vi "Get Module Configuration Example.vi"() -> ()   [LabVIEW 2017]
uses:
  <userlib>/_NEVSTOP/Communicable State Machine(CSM)/_Support/Priority Queue/Priority Queue.lvclass/Priority Queue.ctl
  <userlib>/_NEVSTOP/Communicable State Machine(CSM)/_Support/Process/CSMP-Sync Call.vi
  <userlib>/_NEVSTOP/Communicable State Machine(CSM)/Utility/uuid.vi
  <userlib>/_NEVSTOP/Communicable State Machine(CSM)/Utility/Build Error Cluster.vi
  <userlib>/_NEVSTOP/Communicable State Machine(CSM)/Utility/Trim Both Whitespace.vi
  <userlib>/_NEVSTOP/Communicable State Machine(CSM)/_Support/CSMQ/_CSMObj-Message Check.vi
  <userlib>/_NEVSTOP/Communicable State Machine(CSM)/_Support/CSMQ/_CSMObj-Enqueue Cross-Module Message.vi
  <userlib>/_NEVSTOP/Communicable State Machine(CSM)/_Support/CSMQ/_CSMOFGV Get.vi
  <userlib>/_NEVSTOP/Communicable State Machine(CSM)/_Support/Priority Queue/Enqueue Element.vi
  <userlib>/_NEVSTOP/Communicable State Machine(CSM)/_Support/Error/CSM No Target Error.vi
  <userlib>/_NEVSTOP/Communicable State Machine(CSM)/_Support/CSMQ/_CSMOFGV.vi
  <userlib>/_NEVSTOP/Communicable State Machine(CSM)/_Support/Error/CSM Not Allowed Message.vi
  <userlib>/_NEVSTOP/Communicable State Machine(CSM)/_Support/Error/CSM Target Error.vi
  <userlib>/_NEVSTOP/Communicable State Machine(CSM)/_Support/Error/CSM Unhandled State Error.vi
  <userlib>/_NEVSTOP/Communicable State Machine(CSM)/_Support/Error/CSM Target Timeout Error.vi
  <userlib>/_NEVSTOP/Communicable State Machine(CSM)/Communicable State Machine.lvlib
  API-String-Arugments-Support/API String Arguments Support.lvlib
panel:
  out "Configurations":string[](array[string])
  out "VI Path":path
  out "Core.Current VI Reference":variant
  out "Core.Current VI Reference":string="DoA"
  out "Settings":string="DoA"
  out "error out":errorcluster
  out "DataBool":string="DoA"
  out "DataString":string="DoA"
  out "Settings.Bool":string="DoA"
  out "Settings.String":string="DoA"
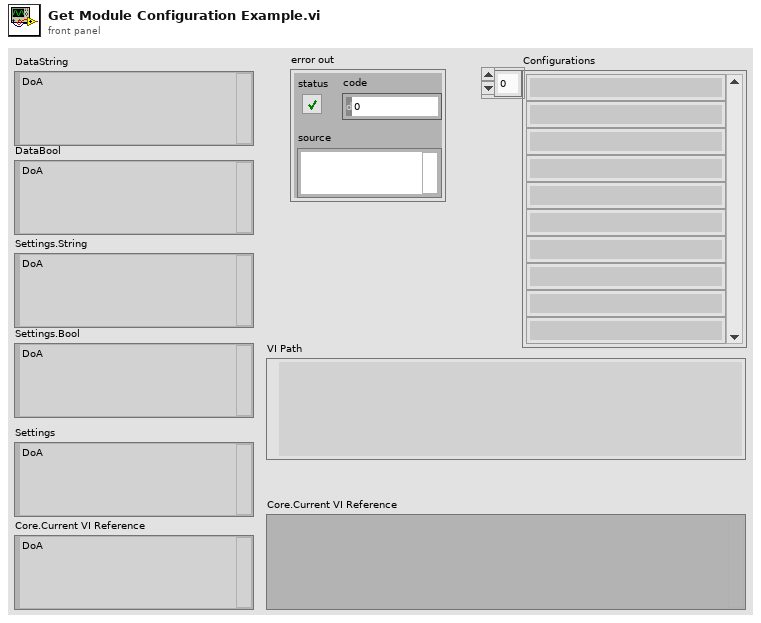
[diagram p1: front panel]
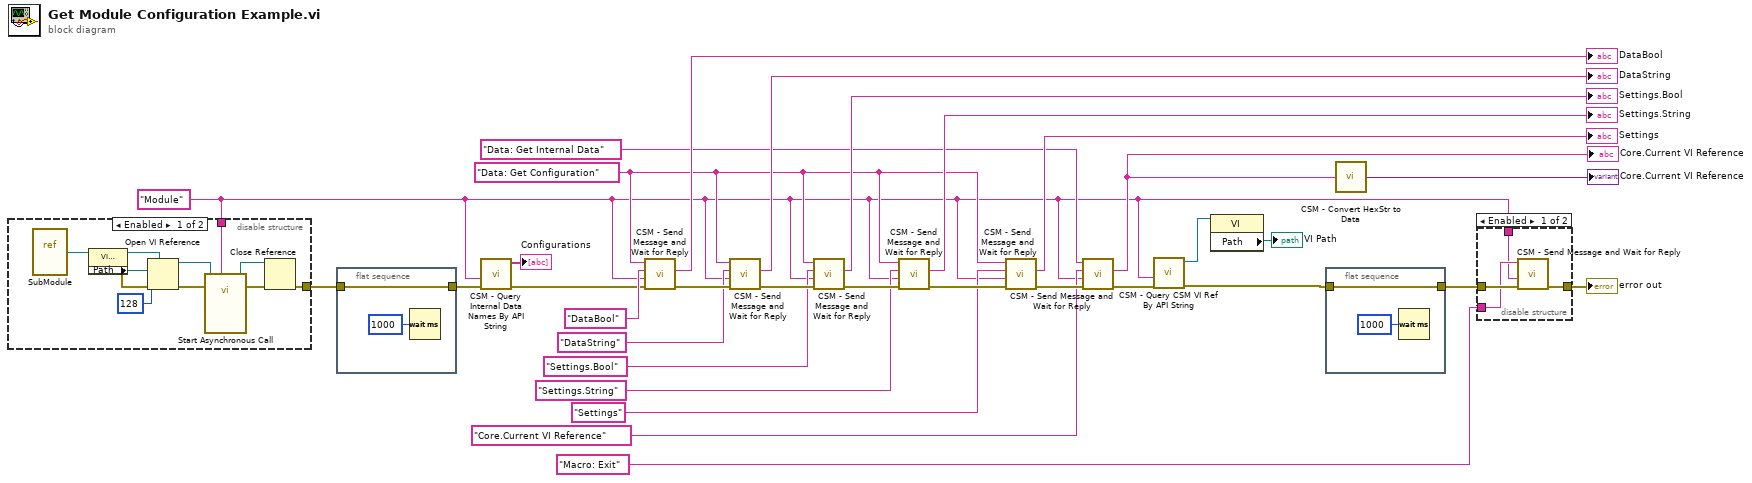
[diagram p0: block diagram]
diagram:
  w17 = "Data: Get Configuration" ("Name(\"\" to use uuid)")
  w1 = "Module" ("Name(\"\" to use uuid)")
  n1 = disable-structure shown="Enabled" {
    disable-tunnel: [w34 _] -> w14
    disable-tunnel: w1 -> [w33 _]
    frame Enabled {
      n2 = vi-ref "SubModule.vi"() -> (w37:refnum<vi>)
      n3 = property class="VI (strict)"(reference=w37) -> (reference out=w41:refnum<vi>, error out=w39:errorcluster, "Path"=w38:path)  [unwired: 1 in]
      n4 = Open VI Reference(type specifier VI Refnum (for type only)=w41, vi path=w38, options=128, error in (no error)=w39) -> (vi reference=w36:refnum<vi>, error out=w42:errorcluster)  [unwired: 2 in]
      n5 = call-by-ref "Start Asynchronous Call"(reference=w36, error in=w42, "Name(\"\" to use uuid)"=w33) -> (reference out=w35:refnum<vi>, error out=w40:errorcluster)  [unwired: 11 in]
      n6 = Close Reference(reference=w35, error in (no error)=w40) -> (error out=w34:errorcluster)
    }
    frame Disabled {
    }
  }
  n7 = flat-sequence {
    tunnel: [w45] -> w4
    tunnel: w14 -> [w45]
    frame #0 {
      n8 = Wait (ms)(milliseconds to wait=u32 1000) -> ()  [unwired: 1 out]
    }
  }
  n9 = call "CSM - Query Internal Data Names By API String.vi"("Error In (no error)"=w4, "Target Module"=w1) -> ("error out"=w3:errorcluster, "Configurations"=→"Configurations":string[])  [unwired: 8 in]
  n10 = call <userlib>:"CSM - Send Message and Wait for Reply.vi"("Error In (no error)"=w3, "Target Module"=w1, "Arguments (\"\")"="DataBool" ("Name(\"\" to use uuid)"), "State"=w17) -> ("error out"=w32:errorcluster, "Response"=→"DataBool":string)  [unwired: 5 in, 1 out]
  n11 = call <userlib>:"CSM - Send Message and Wait for Reply.vi"("Error In (no error)"=w32, "Target Module"=w1, "Arguments (\"\")"="DataString" ("Name(\"\" to use uuid)"), "State"=w17) -> ("error out"=w30:errorcluster, "Response"=→"DataString":string)  [unwired: 5 in, 1 out]
  n12 = call <userlib>:"CSM - Send Message and Wait for Reply.vi"("Error In (no error)"=w30, "Target Module"=w1, "Arguments (\"\")"="Settings.Bool" ("Name(\"\" to use uuid)"), "State"=w17) -> ("error out"=w31:errorcluster, "Response"=→"Settings.Bool":string)  [unwired: 5 in, 1 out]
  n13 = call <userlib>:"CSM - Send Message and Wait for Reply.vi"("Error In (no error)"=w31, "Target Module"=w1, "Arguments (\"\")"="Settings.String" ("Name(\"\" to use uuid)"), "State"=w17) -> ("error out"=w19:errorcluster, "Response"=→"Settings.String":string)  [unwired: 5 in, 1 out]
  n14 = call <userlib>:"CSM - Send Message and Wait for Reply.vi"("Error In (no error)"=w19, "Target Module"=w1, "Arguments (\"\")"="Settings" ("Name(\"\" to use uuid)"), "State"=w17) -> ("error out"=w13:errorcluster, "Response"=→"Settings":string)  [unwired: 5 in, 1 out]
  n15 = call <userlib>:"CSM - Send Message and Wait for Reply.vi"("Error In (no error)"=w13, "Target Module"=w1, "Arguments (\"\")"="Core.Current VI Reference" ("Name(\"\" to use uuid)"), "State"="Data: Get Internal Data" ("Name(\"\" to use uuid)")) -> ("error out"=w8:errorcluster, "Response"=w10:string)  [unwired: 5 in, 1 out]
  "Core.Current VI Reference" <- w10
  n16 = call "CSM - Query CSM VI Ref By API String.vi"("Error In (no error)"=w8, "Target Module"=w1) -> ("error out"=w7:errorcluster, "CSM VI Ref"=w6:refnum<vi>)  [unwired: 8 in]
  n17 = property class="VI"(reference=w6) -> ("Path"=→"VI Path":path)  [unwired: 1 in, 2 out]
  n18 = flat-sequence {
    tunnel: [w47] -> w15
    tunnel: w7 -> [w47]
    frame #0 {
      n19 = Wait (ms)(milliseconds to wait=u32 1000) -> ()  [unwired: 1 out]
    }
  }
  n20 = call <userlib>:"CSM - Convert HexStr to Data.vi"("HEX String"=w10) -> ("Variant"=→"Core.Current VI Reference":variant)  [unwired: 7 in, 1 out]
  n21 = disable-structure shown="Enabled" {
    disable-tunnel: w15 -> [w51 w52]
    disable-tunnel: [w50 w52] -> w21
    disable-tunnel: "Macro: Exit" ("Name(\"\" to use uuid)") -> [w49 _]
    disable-tunnel: w1 -> [w48 _]
    frame Enabled {
      n22 = call <userlib>:"CSM - Send Message and Wait for Reply.vi"("Error In (no error)"=w51, "Target Module"=w48, "State"=w49) -> ("error out"=w50:errorcluster)  [unwired: 6 in, 2 out]
    }
    frame Disabled {
    }
  }
  "error out" <- w21
